vi "MT Generate QAM Synchronization Parameters (number array).vi"(0 "QAM system parameters":T1={"samples per symbol (16)"=16, "symbol map"=[]} {"symbol map" format="%.3f"}, 5 "sync numbers":i32[](array[numeric]) format="%.0x", 7 "bits per sync number":i32=32, 11 "error in (no error)":errorcluster, 12 "expected sync location (symbols)":i32=-1, 13 "sync location uncertainty (symbols)":i32=10, 14 "sync indent (symbols)":i32) -> (4 "QAM synchronization parameters":T2 {"sync sequence" format="%.2f"}, 15 "error out":errorcluster)   [LabVIEW 2020, in "niDMT.lvlib"]
doc: "This polymorphic instance generates synchronization parameters for QAM demodulation using a synchronization sequence defined by a <B>sync numbers</B> array in which each number represents a group of bits."
uses:
  <vilib>/addons/Modulation/niDMT.lvlib
  <vilib>/addons/Modulation/niAMT.lvlib
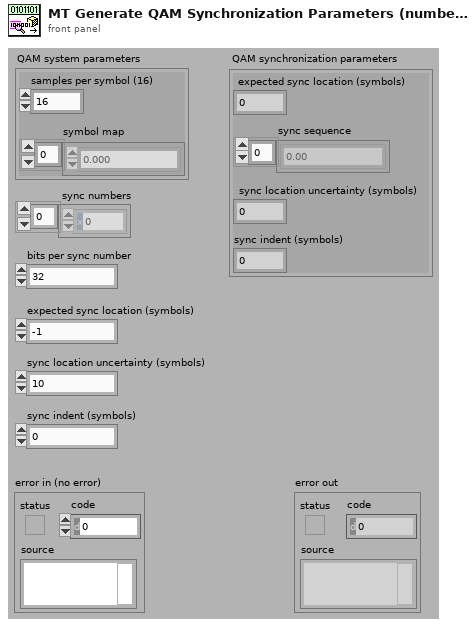
[diagram p1: front panel]
types:
  T1 = cluster{"samples per symbol (16)":i32, "symbol map":cdb[]}
  T2 = cluster{"expected sync location (symbols)":i32, "sync sequence":cdb[], "sync location uncertainty (symbols)":i32, "sync indent (symbols)":i32}
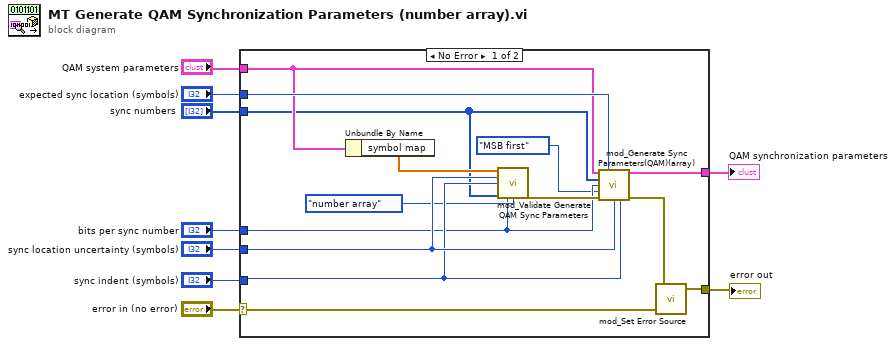
[diagram p0: block diagram]
diagram:
  n1 = case shown="No Error" "error in (no error)" {
    selector: "error in (no error)" -> [w22 w24]
    tunnel: [w20 _] -> w9
    tunnel: "expected sync location (symbols)" -> [w21 _]
    tunnel: "sync location uncertainty (symbols)" -> [w16 _]
    tunnel: "sync indent (symbols)" -> [w15 _]
    tunnel: "sync numbers" -> [w14 _]
    tunnel: "bits per sync number" -> [w11 _]
    tunnel: [w23 w24] -> w2
    tunnel: "QAM system parameters" -> [w18 _]
    frame No Error {
      n2 = Unbundle By Name(w18) -> ("symbol map"=w17:cdb[])
      n3 = call <vilib>:"mod_Validate Generate QAM Sync Parameters.vi"("symbol map"=w17, "sync location uncertainty (symbols)"=w16, "sync indent (symbols)"=w15, "sync numbers"=w14, "number of bits (or) bits per number"=w11, "sync bits specification"=enum16{"bit array", "number array", "number"}."number array") -> ("error out"=w13:errorcluster)  [unwired: 1 in, 8 out]
      n4 = call <vilib>:"mod_Generate Sync Parameters(QAM)(array).vi"("QAM system parameters"=w18, "sync numbers"=w14, "bits per number"=w11, "bit order"=enum16{"MSB first", "LSB first"}."MSB first", "error in (no error)"=w13, "expected sync location (symbols)"=w21, "sync location uncertainty (symbols)"=w16, "sync indent (symbols)"=w15) -> ("QAM synchronization parameters"=w20:T2, "error out"=w19:errorcluster)  [unwired: 6 out]
      n5 = call <vilib>:"mod_Set Error Source.vi"("initial error in (no error)"=w22, "final error in (no error)"=w19) -> ("error out"=w23:errorcluster)  [unwired: 3 out]
    }
    frame Error {
    }
  }
  "QAM synchronization parameters" <- w9
  "error out" <- w2
